vi "TOF.vi"(9 "Delay (ms)":u32=500, 10 "Input":bool) -> (2 "Output":bool)   [LabVIEW 2013]
doc: "The TOF, when given a True input, will immediately output true. When the input reverts back to False, the output will wait for the specified delay to elapse before outputting False."
panel:
  in  "Delay_TOF":T1={"Timer_States"=enum."Input_False_Timing", "Delay-Done_Time"=0}
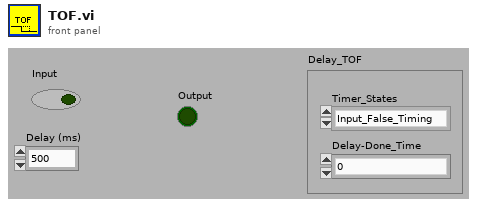
[diagram p1: front panel]
types:
  T1 = cluster{"Timer_States":enum16{"Input_True", "Input_False_Timing", "Input_False_Timing_Complete"}, "Delay-Done_Time":u32}
  T2 = enum16{"Input_True", "Input_False_Timing", "Input_False_Timing_Complete"}
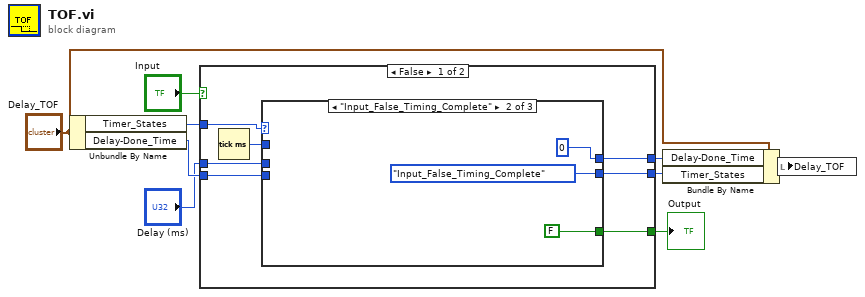
[diagram p0: block diagram]
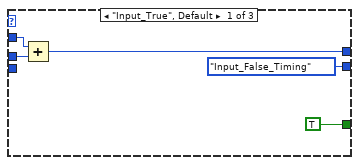
[diagram p2: hidden frame]
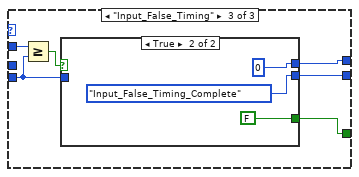
[diagram p3: hidden frame]
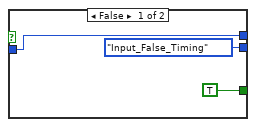
[diagram p4: hidden frame]
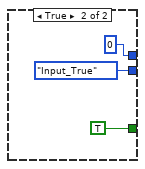
[diagram p5: hidden frame]
diagram:
  n1 = Unbundle By Name("Delay_TOF") -> ("Timer_States"=w5:T2, "Delay-Done_Time"=w8:u32)
  n2 = case shown="False" "Input" {
    tunnel: [w13 TRUE] -> w1
    tunnel: [w14 T2."Input_True" ("Timer_States")] -> w2
    tunnel: [w15 u32 0 ("Delay-Done_Time")] -> w3
    tunnel: w8 -> [w10 _]
    tunnel: w5 -> [w12 _]
    tunnel: "Delay (ms)" -> [w11 _]
    frame False {
      n3 = Tick Count (ms)() -> (millisecond timer value=w16:u32)
      n4 = case shown="\"Input_False_Timing_Complete\"" w12 {
        tunnel: w16 -> [w20 _ w30]
        tunnel: [w18 u32 0 ("Delay-Done_Time") w25] -> w15
        tunnel: [T2."Input_False_Timing" ("Timer_States") T2."Input_False_Timing_Complete" ("Timer_States") w28] -> w14
        tunnel: [TRUE FALSE w27] -> w13
        tunnel: w11 -> [w19 _ _]
        tunnel: w10 -> [_ _ w26]
        frame "Input_True", Default {
          n5 = Add(x=w20, y=w19) -> (x+y=w18:u32)
        }
        frame "Input_False_Timing_Complete" {
        }
        frame "Input_False_Timing" {
          n6 = Greater Or Equal?(x=w30, y=w26) -> (x >= y?=w29:bool)
          n7 = case shown="True" w29 {
            tunnel: [T2."Input_False_Timing" ("Timer_States") T2."Input_False_Timing_Complete" ("Timer_States")] -> w28
            tunnel: [TRUE FALSE] -> w27
            tunnel: w26 -> [w31 _]
            tunnel: [w31 u32 0 ("Delay-Done_Time")] -> w25
            frame False {
            }
            frame True {
            }
          }
        }
      }
    }
    frame True {
    }
  }
  "Output" <- w1
  n8 = Bundle By Name(cluster="Delay_TOF", "Delay-Done_Time"=w3, "Timer_States"=w2) -> (w7:T1)
  n9 = local write "Delay_TOF"(w7) -> ()
